vi "Init UI.vi"(8 "error in (no error)":errorcluster, 11 "Sequencing Control in":refnum<class "Sequencing Control.lvclass">) -> (0 "error out":errorcluster, 3 "Sequencing Control out":refnum<class "Sequencing Control.lvclass">)   [LabVIEW 2020, in "VolatusSeqGUI.lvlib" / "Sequencing Control.lvclass"]
uses:
  Sequencing Control.lvclass
  C:/dev/lv20CE/relink/lv-volatus/VolatusGUI/GUI Element/GUI Element.lvclass
  Colors.ctl
  VolatusGUI/GUI Element/GUI Element.lvclass/GUI Element.ctl
  Sequencing Control.lvclass/Sequencing Control.ctl
  VolatusGUI/GUI Element/GUI Element.lvclass
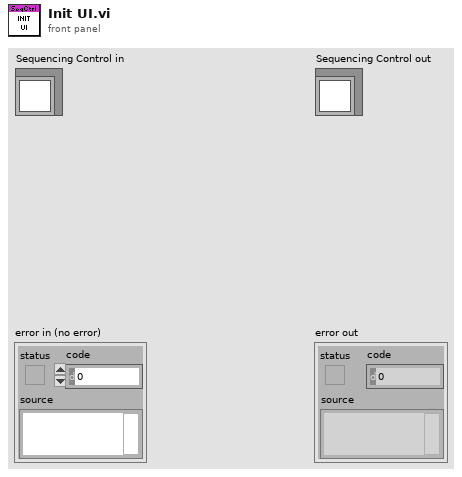
[diagram p1: front panel]
types:
  T1 = typedef "VolatusSeqGUI.lvlib/Sequencing Control.lvclass/Colors.ctl" = cluster{"Default":u32, "Unloaded":u32, "Seq Error":u32, "Loaded Good CRC":u32, "Loaded Bad CRC":u32, "Running Good CRC":u32, "Running Bad CRC":u32}
  T2 = cluster{"[0]":u32, "[1]":u32, "[2]":u32, "[3]":u32, "[4]":u32, "[5]":u32, "[6]":u32}
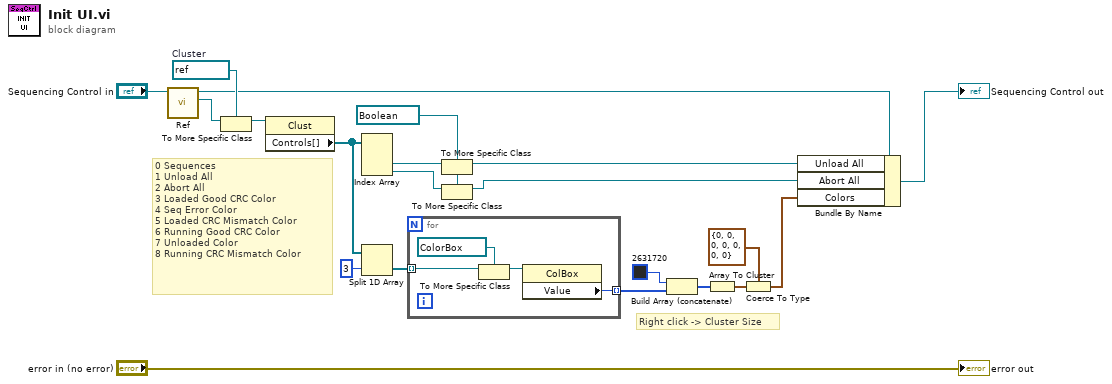
[diagram p0: block diagram]
diagram:
  w16 = refnum<vi> refnum ("Unload All")
  w20 = refnum<vi> refnum  # Cluster
  # "Right click -> Cluster Size"
  # "0 Sequences\n1 Unload All\n2 Abort All\n3 Loaded Good CRC Color\n4 Seq Error Color\n5 Loaded CRC Mismatch Color\n6 Running Good CRC Color\n7 Unloaded Color\n8 Running CRC Mismatch Color"
  n1 = call "Ref.vi"("GUI Element in"="Sequencing Control in") -> ("Ref"=w21:refnum<vi>, "GUI Element out"=w3:refnum<class "Sequencing Control.lvclass">)  [unwired: 9 in]
  n2 = To More Specific Class(target class=w20, reference=w21) -> (specific class reference=w19:refnum<vi>)  [unwired: 1 in, 1 out]
  n3 = property class="Clust"(reference=w19) -> ("Controls[]"=w13:refnum<vi>[])  [unwired: 1 in, 2 out]
  n4 = Index Array(array=w13) -> (element #2=w18:refnum<vi>, element #3=w17:refnum<vi>)  [unwired: 3 in, 1 out]
  n5 = Split 1D Array(array=w13, index=3) -> (second subarray=w11:refnum<vi>[])  [unwired: 1 out]
  n6 = for {
    tunnel: w11 -> [w25] mode=indexing
    tunnel: [w22] -> w10 mode=indexing
    n7 = To More Specific Class(target class=refnum<vi> refnum ("Running, CRC Mismatch"), reference=w25) -> (specific class reference=w23:refnum<vi>)  [unwired: 1 in, 1 out]
    n8 = property class="ColBox"(reference=w23) -> ("Value"=w22:u32)  [unwired: 1 in, 2 out]
  }
  n9 = To More Specific Class(target class=w16, reference=w18) -> (specific class reference=w15:refnum<vi>)  [unwired: 1 in, 1 out]
  n10 = To More Specific Class(target class=w16, reference=w17) -> (specific class reference=w14:refnum<vi>)  [unwired: 1 in, 1 out]
  n11 = Build Array (concatenate)(u32 2631720, w10) -> (w7:u32[])
  n12 = Array To Cluster(array=w7) -> (cluster=w9:T2)
  n13 = Coerce To Type(0:w9, 1:T1 {"Default"=0, "Unloaded"=0, "Seq Error"=0, "Loaded Good CRC"=0, "Loaded Bad CRC"=0, "Running Good CRC"=0, "Running Bad CRC"=0} ("Colors")) -> (2:w5:T1)
  n14 = Bundle By Name(cluster=w3, "Unload All"=w15, "Abort All"=w14, "Colors"=w5) -> (→"Sequencing Control out":refnum<class "Sequencing Control.lvclass">)
  "error out" <- "error in (no error)"
